vi "CheckIntercept.vi"(8 "error in (no error)":errorcluster, 10 "GameRef":refnum<data-value>, 11 "object in":refnum<class "PrimaryAttackerRole.lvclass">) -> (0 "error out":errorcluster, 2 "intercepted":bool, 3 "object out":refnum<class "PrimaryAttackerRole.lvclass">)   [LabVIEW 2023, in "PrimaryAttackerRole.lvclass"]
uses:
  PrimaryAttackerRole.lvclass
  Game_class/Game.lvclass
  Game_class/Game.lvclass/Game.ctl
  Events_class/Events.lvclass/Events.ctl
  Ball_class/Ball.lvclass/Ball.ctl
  Game_class/Read EventsRef.vi
  Game_class/Read BallRef.vi
  Ball_class/Read velocityNorm.vi
  Events_class/Read touch.vi
  Events_class/Read kick.vi
  <vilib>/Analysis/_algsub.llb/Vector Norm.vi
  <vilib>/Analysis/_algsub.llb/Real Vector Norm.vi
  Events_class/Events.lvclass
  Ball_class/Ball.lvclass
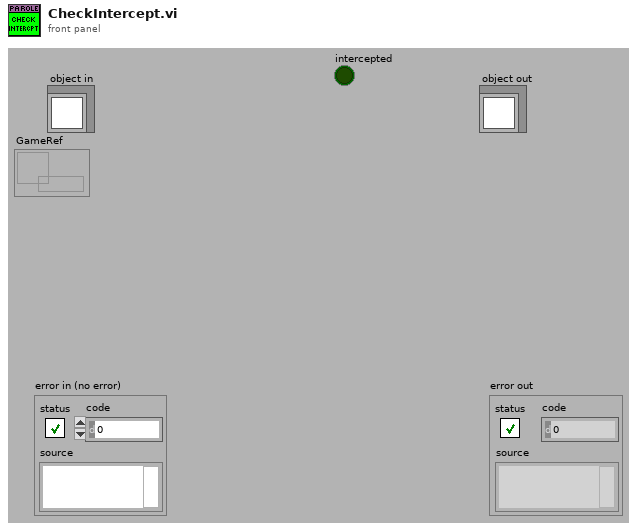
[diagram p1: front panel]
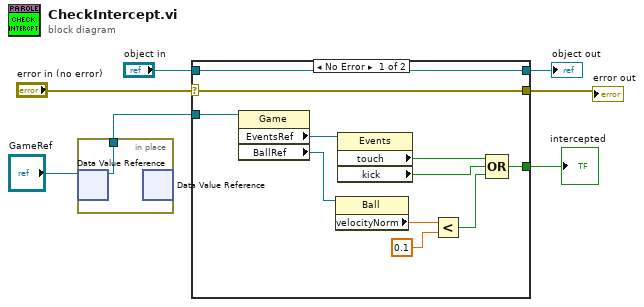
[diagram p0: block diagram]
diagram:
  n1 = in-place {
    in-place-border: [w8] -> w2
    n2 = in-place-dvr #1("GameRef") -> (w8:refnum<class "Game.lvclass">)  [unwired: 1 out]
    n3 = in-place-dvr #1() -> ()  [unwired: 1 in, 2 out]
  }
  n4 = case shown="No Error" "error in (no error)" {
    selector: "error in (no error)" -> [w19 w21]
    tunnel: [w19 w21] -> w6
    tunnel: [w18 w20] -> w4
    tunnel: "object in" -> [w18 w20]
    tunnel: w2 -> [w17 _]
    tunnel: [w9 _] -> w1
    frame No Error {
      n5 = property class="Game"(reference=w17) -> ("EventsRef"=w16:refnum<class "Events.lvclass">, "BallRef"=w15:refnum<class "Ball.lvclass">)  [unwired: 1 in, 2 out]
      n6 = property class="Ball"(reference=w15) -> ("velocityNorm"=w14:dbl)  [unwired: 1 in, 2 out]
      n7 = property class="Events"(reference=w16) -> ("touch"=w12:bool, "kick"=w11:bool)  [unwired: 1 in, 2 out]
      n8 = Less?(x=w14, y=0.1) -> (x < y?=w10:bool)
      n9 = Compound Arithmetic op=OR(w12, w11, w10) -> (w9:bool)
    }
    frame Error {
    }
  }
  "error out" <- w6
  "object out" <- w4
  "intercepted" <- w1
